vi "new hexidecimal.vi"(10 "Numeric":u8 max=15 format="%x") -> (2 "display":T1)   [LabVIEW 2009]
uses:
  display.ctl
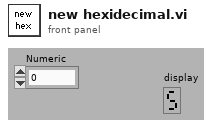
[diagram p1: front panel]
types:
  T1 = typedef "display.ctl" = cluster{"LED 0":bool, "LED 1":bool, "LED 2":bool, "LED 4":bool, "LED 8":bool}
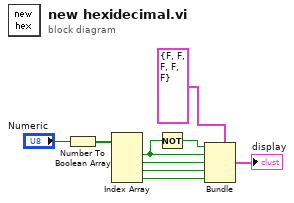
[diagram p0: block diagram]
diagram:
  n1 = Number To Boolean Array(number="Numeric") -> (Boolean array=w7:bool[])
  n2 = Index Array(array=w7) -> (element #1=w5:bool, element #2=w4:bool, element #3=w3:bool, element #4=w2:bool)  [unwired: 4 in]
  n3 = Not(x=w5) -> (.not. x?=w6:bool)
  n4 = Bundle(cluster=T1 {"LED 0"=FALSE, "LED 1"=FALSE, "LED 2"=FALSE, "LED 4"=FALSE, "LED 8"=FALSE} ("display"), "LED 0"=w6, "LED 1"=w5, "LED 2"=w4, "LED 4"=w3, "LED 8"=w2) -> (→"display":T1)
